vi "lowpass_derivative_with_filter.vi"(9 "sigma_time":dbl=10.0 format="%#_13g", 10 "sampling frequency":dbl=0.1, 11 "X":dbl[](array[numeric])) -> (3 "dX":dbl[](array[numeric]))   [LabVIEW 2017]
uses:
  <vilib>/Analysis/2dsp.llb/1D Convolution (DBL).vi
  <vilib>/Analysis/NI_AALPro.lvlib
panel:
  out "change":dbl
  out "int of deriv":dbl
  out "sum":dbl
  out "input size":i32
  out "kernel size":i32
  out "Y":dbl[](graph)
  out "pad size":i32
  out "conv size":i32
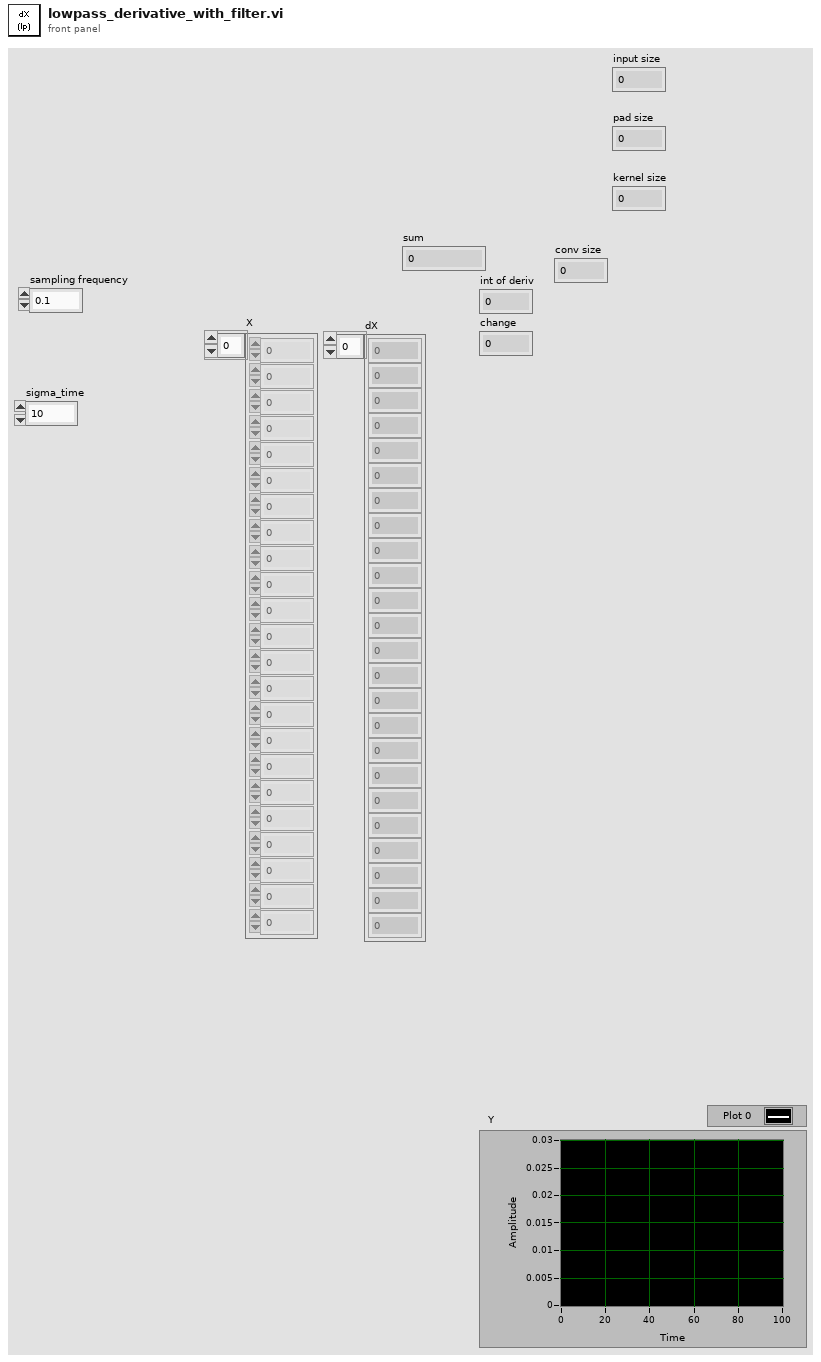
[diagram p1: front panel]
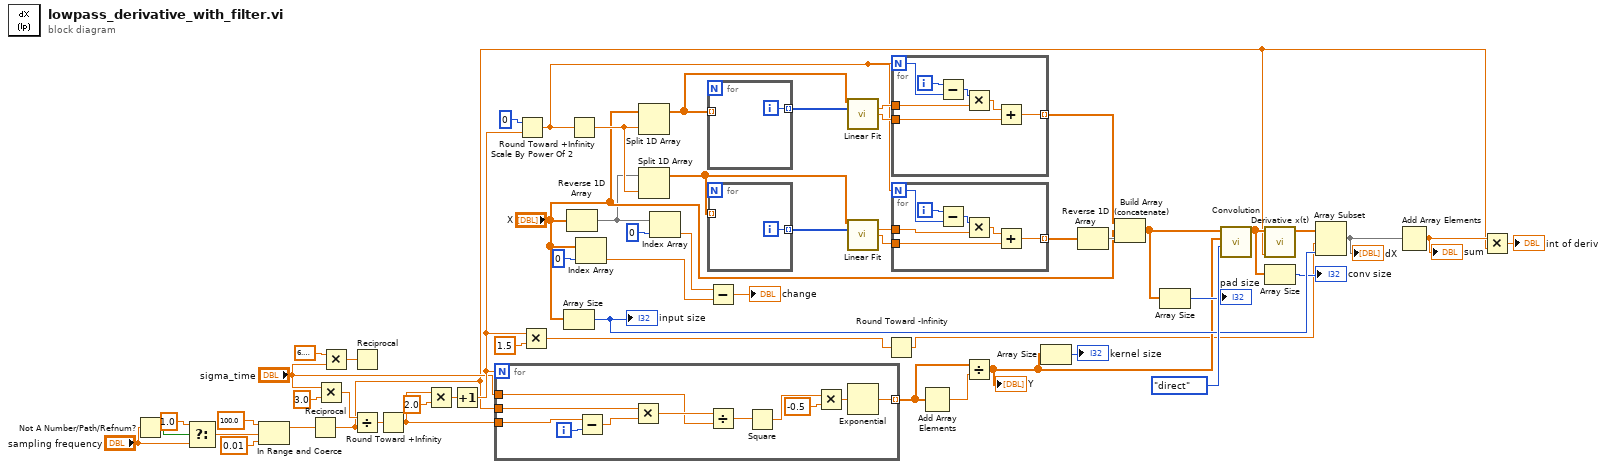
[diagram p0: block diagram]
diagram:
  n1 = Not A Number/Path/Refnum?(number/path/refnum="sampling frequency") -> (NaN/Path/Refnum?=w44:bool)
  n2 = Select(t=1.0, s=w44, f="sampling frequency") -> (s? t:f=w41:dbl)
  n3 = In Range and Coerce(upper limit=100.0, x=w41, lower limit=0.01) -> (coerced(x)=w47:dbl)  [unwired: 1 out]
  n4 = Reciprocal(x=w47) -> (1/x=w8:dbl)
  n5 = Multiply(x="sigma_time", y=3.0) -> (x*y=w53:dbl)
  n6 = Multiply(x=6.283185307179586, y="sigma_time") -> (x*y=w55:dbl)
  n7 = Reciprocal(x=w55) -> ()  [unwired: 1 out]
  n8 = Divide(x=w53, y=w8) -> (x/y=w52:dbl)
  n9 = Round Toward +Infinity(x=w52) -> (ceil(x): smallest int >= x=w5:dbl)
  n10 = Multiply(x=w5, y=2.0) -> (x*y=w13:dbl)
  n11 = Increment(x=w13) -> (x+1=w14:dbl)
  n12 = for {
    N: w14 -> [_]
    tunnel: w5 -> [w67]
    tunnel: w8 -> [w64]
    tunnel: "sigma_time" -> [w62]
    tunnel: [w57] -> w11 mode=indexing
    i -> [w66]
    n13 = Subtract(x=w67, y=w66) -> (x-y=w65:dbl)
    n14 = Multiply(x=w64, y=w65) -> (x*y=w63:dbl)
    n15 = Divide(x=w63, y=w62) -> (x/y=w61:dbl)
    n16 = Square(x=w61) -> (x^2=w60:dbl)
    n17 = Multiply(x=w60, y=-0.5) -> (x*y=w58:dbl)
    n18 = Exponential(1:w58) -> (0:w57:dbl)
  }
  n19 = Scale By Power Of 2(n=i16 0, x=w14) -> (x*2^n=w24:dbl)
  n20 = Multiply(x=w14, y=1.5) -> (x*y=w3:dbl)
  n21 = Array Size(array="X") -> (size(s)=w48:i32)
  "input size" <- w48
  n22 = Reverse 1D Array(array="X") -> (reversed array=w19:dbl[])
  n23 = Round Toward +Infinity(x=w24) -> (ceil(x): smallest int >= x=w30:dbl)
  n24 = Index Array(array="X", index=0) -> (element=w16:dbl)
  n25 = Split 1D Array(array="X", index=w30) -> (first subarray=w26:dbl[])  [unwired: 1 out]
  n26 = Split 1D Array(array=w19, index=w30) -> (first subarray=w29:dbl[])  [unwired: 1 out]
  n27 = Index Array(array=w19, index=0) -> (element=w17:dbl)
  n28 = for {
    tunnel: [w68] -> w37 mode=indexing
    tunnel: w26 -> [_] mode=indexing
    i -> [w68]
  }
  n29 = for {
    tunnel: [w69] -> w33 mode=indexing
    tunnel: w29 -> [_] mode=indexing
    i -> [w69]
  }
  n30 = Subtract(x=w17, y=w16) -> (x-y=→"change":dbl)
  n31 = call <vilib>:"Linear Fit.vi"("Y"=w26, "X"=w37) -> ("slope"=w36:dbl, "intercept"=w35:dbl)  [unwired: 9 in, 3 out]
  n32 = call <vilib>:"Linear Fit.vi"("Y"=w29, "X"=w33) -> ("slope"=w32:dbl, "intercept"=w31:dbl)  [unwired: 9 in, 3 out]
  n33 = Round Toward -Infinity(1:w3) -> (0:w1:dbl)
  n34 = for {
    N: w24 -> [w75]
    tunnel: w36 -> [w73]
    tunnel: w35 -> [w71]
    tunnel: [w70] -> w34 mode=indexing
    i -> [w76]
    n35 = Subtract(x=w76, y=w75) -> (x-y=w74:i32)
    n36 = Multiply(x=w74, y=w73) -> (x*y=w72:dbl)
    n37 = Add(x=w72, y=w71) -> (x+y=w70:dbl)
  }
  n38 = for {
    N: w24 -> [w82]
    tunnel: w32 -> [w80]
    tunnel: w31 -> [w78]
    tunnel: [w77] -> w28 mode=indexing
    i -> [w83]
    n39 = Subtract(x=w83, y=w82) -> (x-y=w81:i32)
    n40 = Multiply(x=w81, y=w80) -> (x*y=w79:dbl)
    n41 = Add(x=w79, y=w78) -> (x+y=w77:dbl)
  }
  n42 = Add Array Elements(numeric array=w11) -> (sum=w10:dbl)
  n43 = Divide(x=w11, y=w10) -> (x/y=w6:dbl[])
  "Y" <- w6
  n44 = Array Size(array=w6) -> (size(s)=→"kernel size":i32)
  n45 = Reverse 1D Array(array=w28) -> (reversed array=w27:dbl[])
  n46 = Build Array (concatenate)(w34, "X", w27) -> (w4:dbl[])
  n47 = Array Size(array=w4) -> (size(s)=→"pad size":i32)
  n48 = call-poly <vilib>:"Convolution.vi"("algorithm"=enum32{"direct", "frequency domain"}."direct", "Y"=w6, "X"=w4) -> ("X * Y"=w9:dbl[])  [unwired: 7 in, 1 out]
  n49 = call <vilib>:"Derivative x(t).vi"("dt"=w8, "X"=w9) -> ("dX/dt"=w7:dbl[])  [unwired: 8 in, 1 out]
  n50 = Array Size(array=w9) -> (size(s)=→"conv size":i32)
  n51 = Array Subset(array=w7, index=w1, length=w48) -> (w22:dbl[])
  "dX" <- w22
  n52 = Add Array Elements(numeric array=w22) -> (sum=w21:dbl)
  "sum" <- w21
  n53 = Multiply(x=w21, y=w8) -> (x*y=→"int of deriv":dbl)
